vi "Define Mapping Column.vi"(4 "DT Dependency":i32=-1, 5 "Read Only (F)":bool, 6 "data type":T2, 7 "Call Back VI":T1, 8 "name dependency":i32=-1, 9 "Channel suffix":string, 10 "caption":string, 11 "name":string) -> (2 "Column Descriptor out":T3={"name"="Link", "caption"="", "Column Type"=enum."String", "Params"="", "AutoSizeMode"=1, "FillWeight"=100.0, "MinWidth"=50, "tooltip"="The quick brown fox jumps over the lazy dog", "Enum Reference"=refnum, "Channel suffix"="", "Read Only"=FALSE, "Call Back VI"=refnum, "DT Dependency"=0, "name dependency"=0, "data type"=enum."Double", "Custom Column"=refnum} {"MinWidth" min=2 step=1; "AutoSizeMode" items=["None"=1, "ColumnHeader"=2, "AllCellsExceptHeader"=4, "AllCells"=6, "DisplayedCellsExceptHeader"=8, "DisplayedCells"=10, "Fill"=16]; "FillWeight" min=1 max=100})   [LabVIEW 2013, in "Table Manager.lvlib" / "Mapping Column.lvclass"]
doc: "This VI describes a 'mapping column' that will map a channel to a tag. \nThe name of the channel is built concatenating the name dependecy column value with the channel suffix. The datatype will be the value of the column indicated in DT dependecy if its (-1) it will use the Datatype control."
uses:
  Mapping Column.lvclass
  Column/Column Descriptor.ctl
  Column/Column.lvclass
  Column/Column Type.ctl
  <vilib>/NI/Tag Bus/tag/Data Type.ctl
  Table Manager/Call Back Ref Type Def.ctl
  Configuration Editor/Classes/Engine Parent/Engine Parent Editor Node.lvclass
  Configuration Editor/Classes/Module editor node/module editor node.lvclass
  <vilib>/NI/Tag Bus/tag/tag descriptor.lvclass
  Table Manager/Table Manager.lvclass
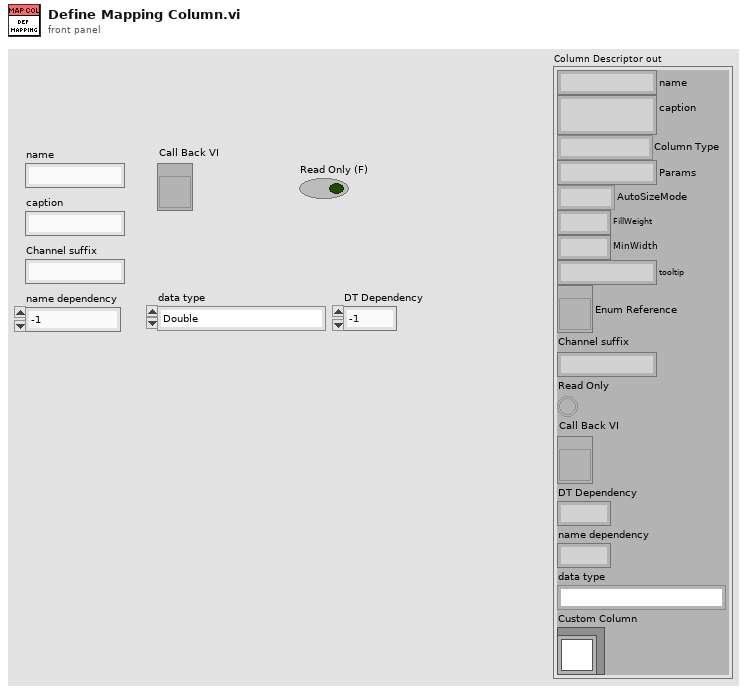
[diagram p1: front panel]
types:
  T1 = typedef "Table Manager.lvlib/Table Manager.lvclass/Call Back Ref Type Def.ctl" = refnum<vi>
  T2 = typedef "tag bus.lvlib/tag descriptor.lvclass/Data Type.ctl" = enum16{"Double", "Single", "I64", "I32", "I16", "I8", "U64", "U32", "U16", "U8", "Boolean", "String", "Array of Double", "Array of Single", "Array of I64", "Array of I32", "Array of I16", "Array of I8", "Array of U64", "Array of U32", "Array of U16", "Array of U8", "Array of Boolean", "Array of String"}
  T3 = typedef "Table Manager.lvlib/Column.lvclass/Column Descriptor.ctl" = cluster{"name":string, "caption":string, "Column Type":T4, "Params":string, "AutoSizeMode":i32, "FillWeight":sgl, "MinWidth":u32, "tooltip":string, "Enum Reference":refnum<vi>, "Channel suffix":string, "Read Only":bool, "Call Back VI":T1, "DT Dependency":i32, "name dependency":i32, "data type":T2, "Custom Column":refnum<class "Column.lvclass">}
  T4 = typedef "Table Manager.lvlib/Column.lvclass/Column Type.ctl" = enum16{"String", "Mapping", "Enum", "Custom"}
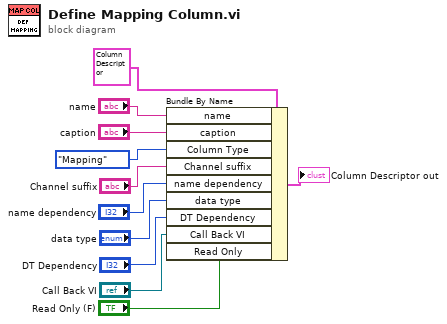
[diagram p0: block diagram]
diagram:
  n1 = Bundle By Name(cluster=T3 {"name"="", "caption"="", "Column Type"=enum."String", "Params"="", "AutoSizeMode"=16, "FillWeight"=100.0, "MinWidth"=50, "tooltip"="", "Enum Reference"=refnum, "Channel suffix"="", "Read Only"=FALSE, "Call Back VI"=refnum, "DT Dependency"=0, "name dependency"=0, "data type"=enum."Double", "Custom Column"=refnum} ("Table Manager.lvlib:Column.lvclass:Column Descriptor"), "name"="name", "caption"="caption", "Column Type"=Column_Type."Mapping", "Channel suffix"="Channel suffix", "name dependency"="name dependency", "data type"="data type", "DT Dependency"="DT Dependency", "Call Back VI"="Call Back VI", "Read Only"="Read Only (F)") -> (→"Column Descriptor out":T3)
